vi "rad_Apply Network Settings (DHCP).vi"(8 "error in (no error)":errorcluster, 10 "Requested settings":T1={"Hostname"="", "Serial number"="", "Product name"="", "Product code"=0, "System status"="", "Credential type"=enum."None/Unlocked", "User added?"=FALSE, "Primary NIC"={"MAC address"="", "IP Address Request Mode"=2, "IP address"="", "Subnet mask"="", "Gateway"="", "DNS server"=""}} {"Primary NIC"."IP Address Request Mode" items=["Static"=1, "DHCP/Link-Local"=2, "Link-Local Only"=4, "DHCP Only"=8]}, 11 "Existing settings":T1={"Hostname"="", "Serial number"="", "Product name"="", "Product code"=0, "System status"="", "Credential type"=enum."None/Unlocked", "User added?"=FALSE, "Primary NIC"={"MAC address"="", "IP Address Request Mode"=2, "IP address"="", "Subnet mask"="", "Gateway"="", "DNS server"=""}} {"Primary NIC"."IP Address Request Mode" items=["Static"=1, "DHCP/Link-Local"=2, "Link-Local Only"=4, "DHCP Only"=8]}) -> (0 "error out":errorcluster, 3 "Target settings out":T1={"Hostname"="", "Serial number"="", "Product name"="", "Product code"=0, "System status"="", "Credential type"=enum."None/Unlocked", "User added?"=FALSE, "Primary NIC"={"MAC address"="", "IP Address Request Mode"=2, "IP address"="", "Subnet mask"="", "Gateway"="", "DNS server"=""}} {"Primary NIC"."IP Address Request Mode" items=["Static"=1, "DHCP/Link-Local"=2, "Link-Local Only"=4, "DHCP Only"=8]})   [LabVIEW 2016]
uses:
  TypeDefs/rad_Target Information.ctl
  TypeDefs/rad_Target Network Settings.ctl
  rad_Globals.vi
  <vilib>/nisyscfg/Save Changes (System).vi
  <vilib>/nisyscfg/Close (System).vi
  <vilib>/nisyscfg/nisyscfg.lvlib
  <resource>/objmgr/nisysapi.rc
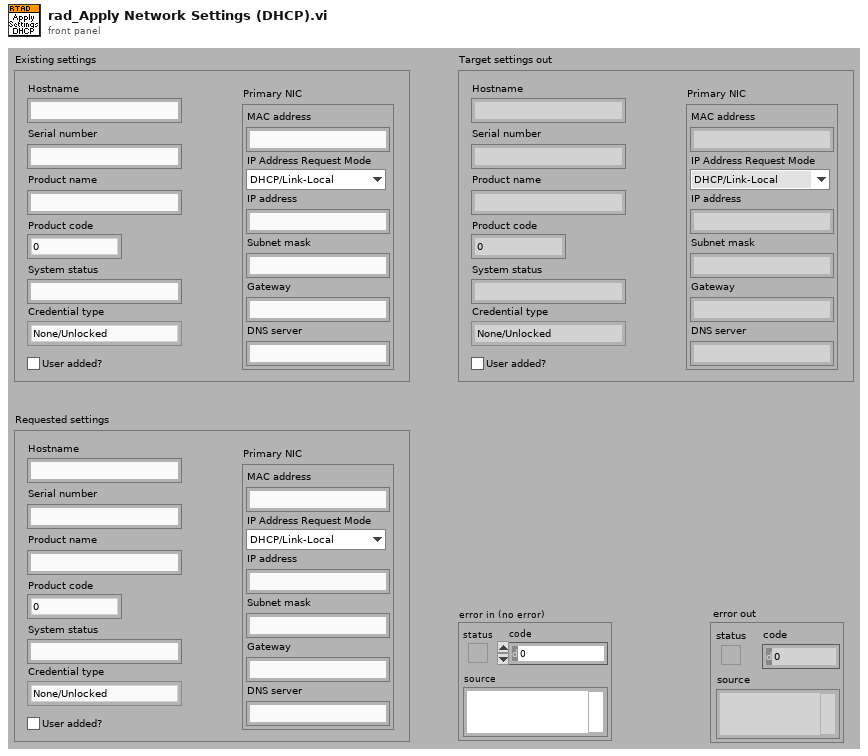
[diagram p1: front panel]
types:
  T1 = typedef "rad_Target Information.ctl" = cluster{"Hostname":string, "Serial number":string, "Product name":string, "Product code":i32, "System status":string, "Credential type":enum16{"None/Unlocked", "FTP Password", "NIAuth Credentials"}, "User added?":bool, "Primary NIC":T2}
  T2 = typedef "rad_Target Network Settings.ctl" = cluster{"MAC address":string, "IP Address Request Mode":i32, "IP address":string, "Subnet mask":string, "Gateway":string, "DNS server":string}
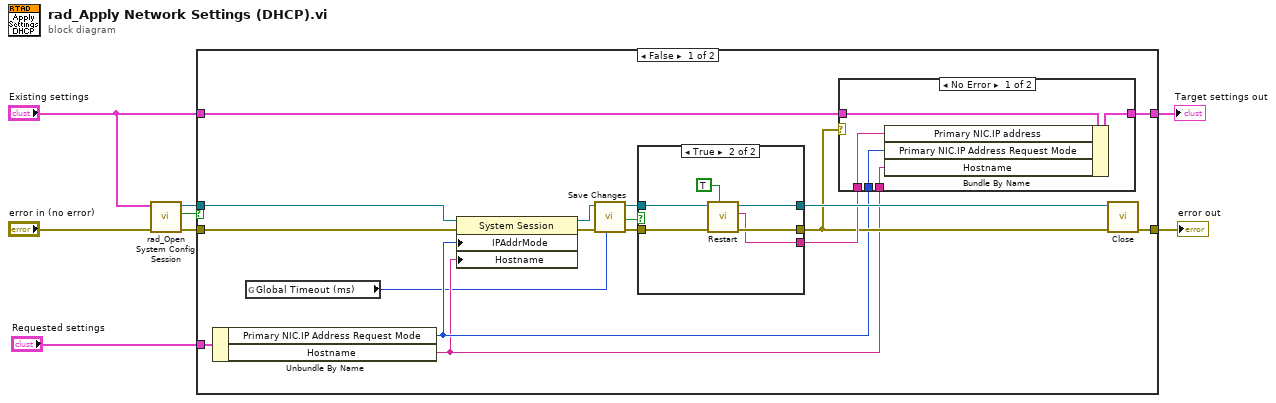
[diagram p0: block diagram]
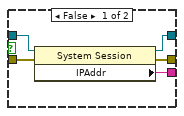
[diagram p3: hidden frame]
diagram:
  n1 = call "rad_Open System Config Session.vi"("error in (no error)"="error in (no error)", "Target settings"="Existing settings") -> ("error out"=w5:errorcluster, "Cancelled"=w4:bool, "Session out"=w6:refnum<k21>)  [unwired: 6 in, 1 out]
  n2 = case shown="False" w4 {
    tunnel: w6 -> [w25 _]
    tunnel: w5 -> [w24 w44]
    tunnel: [w23 w44] -> w7
    tunnel: "Existing settings" -> [w17 w43]
    tunnel: [w16 w43] -> w3
    tunnel: "Requested settings" -> [w12 _]
    frame False {
      n3 = Unbundle By Name(w12) -> ("Primary NIC.IP Address Request Mode"=w11:i32, "Hostname"=w10:string)
      n4 = global read "rad_Globals.vi" "Global Timeout (ms)"() -> (w9:u32)
      n5 = property class="System Session"(reference=w25, error in=w24, "IPAddrMode"=w11, "Hostname"=w10) -> (reference out=w22:refnum<k21>, error out=w21:errorcluster)
      n6 = call-poly <vilib>:"Save Changes.vi"("Remote Timeout (300,000 ms)"=w9, "error in (no error)"=w21, "Session in"=w22) -> ("error out"=w19:errorcluster, "Changes Require Restart"=w20:bool, "Session out"=w18:refnum<k21>)  [unwired: 5 in, 1 out]
      n7 = case shown="True" w20 {
        tunnel: w19 -> [w36 w42]
        tunnel: [w35 w41] -> w13
        tunnel: w18 -> [w34 w40]
        tunnel: [w33 w39] -> w15
        tunnel: [w32 w37] -> w14
        frame False {
          n8 = property class="System Session"(reference=w34, error in=w36) -> (reference out=w33:refnum<k21>, error out=w35:errorcluster, "IPAddr"=w32:string)
        }
        frame True {
          n9 = call <vilib>:"Restart.vi"("Wait Until Complete (T)"=TRUE ("wait until complete (T)"), "error in (no error)"=w42, "Session in"=w40) -> ("error out"=w41:errorcluster, "New IP Address"=w37:string, "Session out"=w39:refnum<k21>)  [unwired: 6 in]
        }
      }
      n10 = case shown="No Error" w13 {
        tunnel: w17 -> [w30 w31]
        tunnel: [w29 w31] -> w16
        tunnel: w10 -> [w28 _]
        tunnel: w11 -> [w27 _]
        tunnel: w14 -> [w26 _]
        frame No Error {
          n11 = Bundle By Name(cluster=w30, "Primary NIC.IP address"=w26, "Primary NIC.IP Address Request Mode"=w27, "Hostname"=w28) -> (w29:T1)
        }
        frame Error {
        }
      }
      n12 = call-poly <vilib>:"Close.vi"("error in (no error)"=w13, "Session in"=w15) -> ("error out"=w23:errorcluster)  [unwired: 9 in]
    }
    frame True {
    }
  }
  "error out" <- w7
  "Target settings out" <- w3
